vi "Set Turbo Valve DAC.vi"(10 "IILCDAC":refnum<class "ILC DAC.lvclass">, 11 "ILC Actuator Cylinder in":refnum<class "ILC Actuator Cylinder.lvclass">) -> (3 "ILC Actuator Cylinder out":refnum<class "ILC Actuator Cylinder.lvclass">)   [LabVIEW 2015, in "ILC Actuator Cylinder.lvclass"]
uses:
  ILC Actuator Cylinder.lvclass
  ILC DAC/ILC DAC/ILC DAC.lvclass
  ILC Actuator Cylinder.lvclass/ILC Actuator Cylinder.ctl
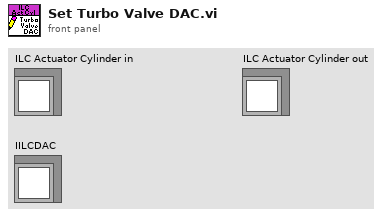
[diagram p1: front panel]
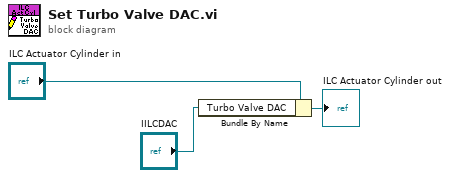
[diagram p0: block diagram]
diagram:
  n1 = Bundle By Name(cluster="ILC Actuator Cylinder in", "Turbo Valve DAC"="IILCDAC") -> (→"ILC Actuator Cylinder out":refnum<class "ILC Actuator Cylinder.lvclass">)
